vi "CollisionDetection_main.vi"(0 "Image In":T1, 5 "Collision\nDetection":bool, 7 "Overlay":bool, 11 "Error In":errorcluster, 12 "Laser Detected Old":bool) -> (3 "Collision Detected":bool, 4 "Image Out":T1, 6 "Distance to Wall (m)":dbl, 8 "Perpendicular Distance to Wall (m)":dbl, 10 "delta° (incident angle)":dbl, 13 "Laser Detected":bool, 14 "Laser Detected Twice":bool, 15 "Error Out":errorcluster)   [LabVIEW 2013]
uses:
  <vilib>/vision/Image Controls.llb/IMAQ Image.ctl
panel:
  out "Intensity":cluster{u8[], i32[]}[](graph)
  in  "F = Gauss S\nT = Gauss ES":bool
  in  "F = I_max\nT = Gauss":bool
  in  "index":i32
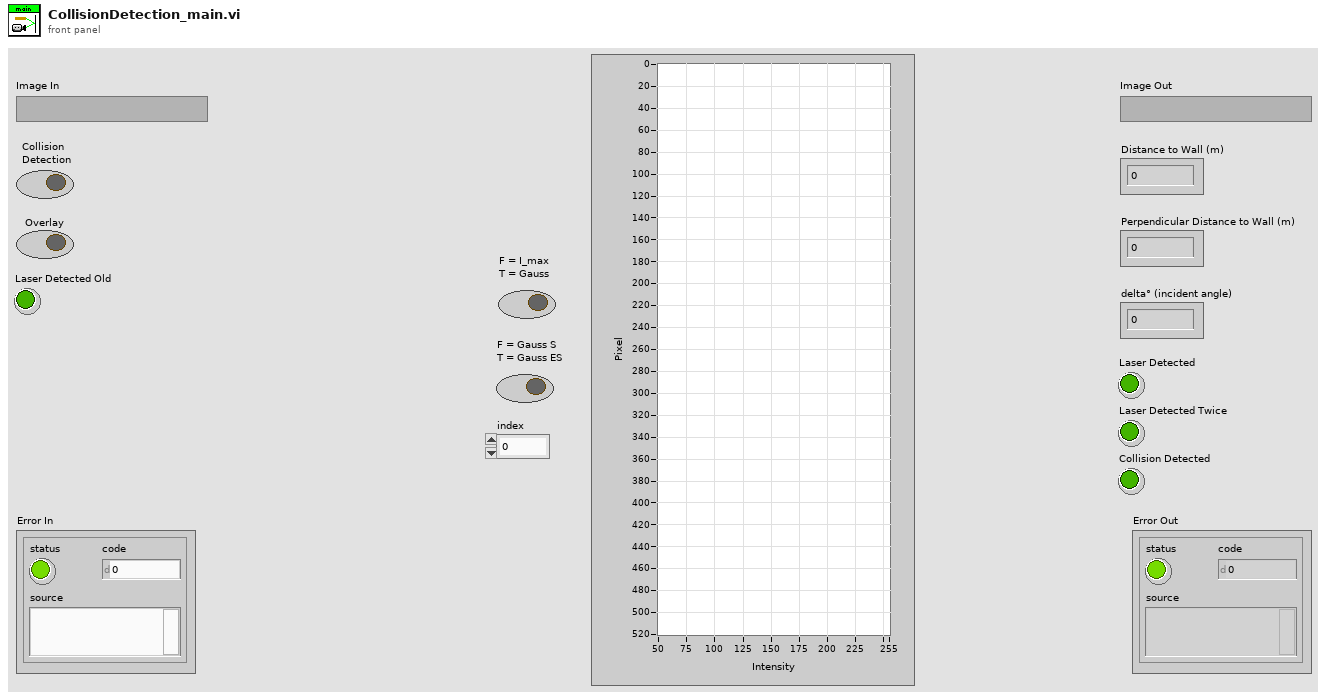
[diagram p1: front panel]
types:
  T1 = typedef "IMAQ Image.ctl" = refnum<image>
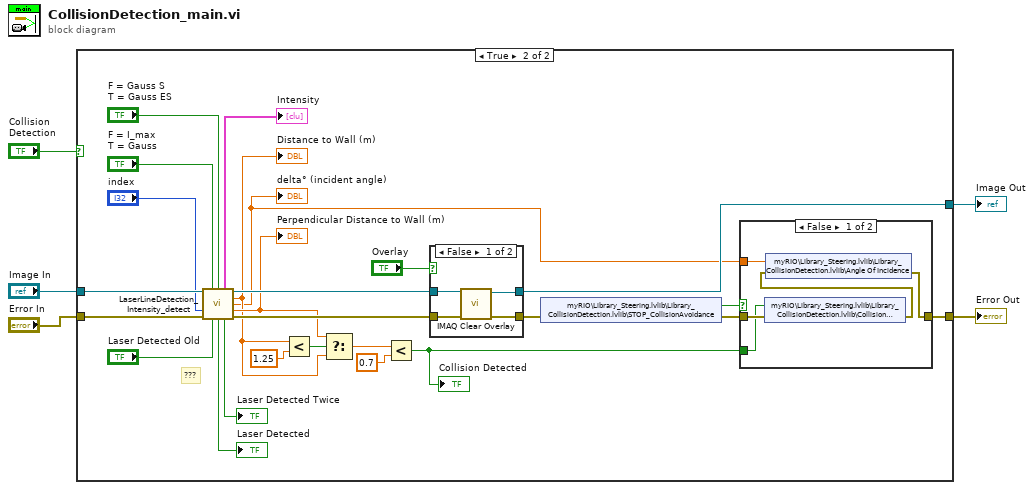
[diagram p0: block diagram]
diagram:
  n1 = case shown="True" "Collision\nDetection" {
    tunnel: "Error In" -> [w6 w26]
    tunnel: [w6 w32] -> w4
    tunnel: [w7 w31] -> w2
    tunnel: "Image In" -> [w7 w24]
    frame False {
    }
    frame True {
      # "???"
      n2 = call "LaserLineDetection_Intensity_detect.vi"("Source In"=w24, "F = I_max\nT = Gauss"="F = I_max\nT = Gauss", "F = Gauss S\nT = Gauss ES"="F = Gauss S\nT = Gauss ES", "index"="index", "Error In"=w26, "Laser Detected Old"="Laser Detected Old") -> ("appended array"=→"Intensity":cluster{u8[], i32[]}[], "Source Out"=w23:T1, "Distance to Wall (m)"=w9:dbl, "delta° (incident angle)"=w8:dbl, "Perpendicular Distance to Wall (m)"=w10:dbl, "Laser Detected"=→"Laser Detected":bool, "Laser Detected Twice"=→"Laser Detected Twice":bool, "Error Out"=w25:errorcluster)  [unwired: 2 in]
      "Distance to Wall (m)" <- w9
      "Perpendicular Distance to Wall (m)" <- w10
      "delta° (incident angle)" <- w8
      n3 = Less?(x=w9, y=1.25) -> (x < y?=w22:bool)
      n4 = Select(t=w10, s=w22, f=w9) -> (s? t:f=w20:dbl)
      n5 = Less?(x=w20, y=0.7) -> (x < y?=w11:bool)
      "Collision Detected" <- w11
      n6 = case shown="False" "Overlay" {
        tunnel: [w42 w44] -> w28
        tunnel: w25 -> [w41 w44]
        tunnel: [w40 w43] -> w31
        tunnel: w23 -> [w39 w43]
        frame False {
          n7 = call "IMAQ Clear Overlay"("error in (no error)"=w41, "Image"=w39) -> ("error out"=w42:errorcluster, "Image Out"=w40:T1)  [unwired: 8 in]
        }
        frame True {
        }
      }
      n8 = shared-variable "myRIO\\Library_Steering.lvlib\\Library_CollisionDetection.lvlib\\STOP_CollisionAvoidance"(error in=w28) -> (w29:bool, error out=w27:errorcluster)
      n9 = case shown="False" w29 {
        tunnel: [w33 w38] -> w32
        tunnel: w27 -> [w37 w38]
        tunnel: w11 -> [w36 _]
        tunnel: w8 -> [w35 _]
        frame False {
          n10 = shared-variable "myRIO\\Library_Steering.lvlib\\Library_CollisionDetection.lvlib\\Collision Detected"(w36, error in=w37) -> (error out=w34:errorcluster)
          n11 = shared-variable "myRIO\\Library_Steering.lvlib\\Library_CollisionDetection.lvlib\\Angle Of Incidence"(w35, error in=w34) -> (error out=w33:errorcluster)
        }
        frame True {
        }
      }
    }
  }
  "Error Out" <- w4
  "Image Out" <- w2
